vi "Read Test Information.vi"(8 "error in (no error)":errorcluster, 11 "Results List in":refnum<class "Results List.lvclass">) -> (0 "error out":errorcluster, 2 "Test Information":T1, 3 "Results List out":refnum<class "Results List.lvclass">)   [LabVIEW 2015, in "Results List.lvclass"]
uses:
  Results List.lvclass
  Test Information.ctl
  Results List.lvclass/Results List.ctl
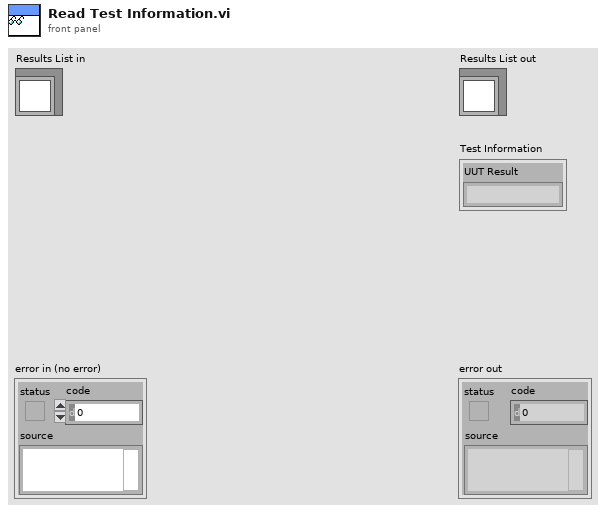
[diagram p1: front panel]
types:
  T1 = typedef "Results List.lvclass/Test Information.ctl" = cluster{"UUT Result":string}
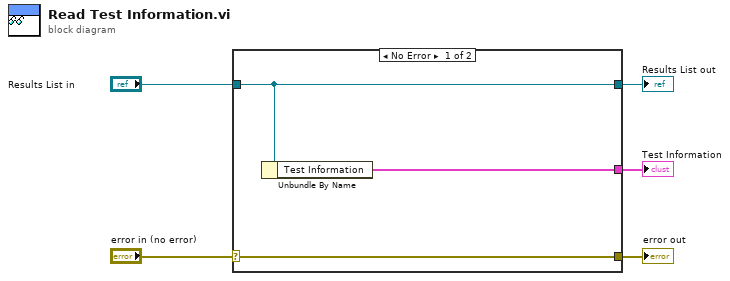
[diagram p0: block diagram]
diagram:
  n1 = case shown="No Error" "error in (no error)" {
    selector: "error in (no error)" -> [w8 w9]
    tunnel: [w8 w9] -> w4
    tunnel: [w7 w10] -> w2
    tunnel: "Results List in" -> [w7 w10]
    tunnel: [w6 _] -> w1
    frame No Error {
      n2 = Unbundle By Name(w7) -> ("Test Information"=w6:T1)
    }
    frame Error {
    }
  }
  "error out" <- w4
  "Results List out" <- w2
  "Test Information" <- w1
